vi "Clear Attachments2.vi"(0 "handles cluster in":T1 caption="ハンドルクラスター入力", 11 "error in (no error)":errorcluster caption="エラー入力（エラーなし）") -> (4 "handles cluster out":T1 caption="ハンドルクラスター出力", 15 "error out":errorcluster caption="エラー出力")   [LabVIEW 2015]
doc: "「Set Attachments2」VIを使用して設定したすべての添付を除去します。"
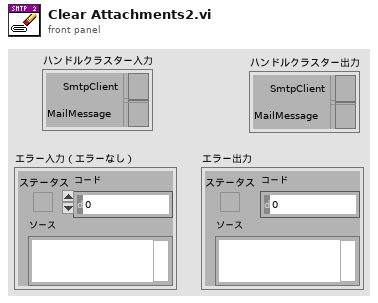
[diagram p1: front panel]
types:
  T1 = cluster{"SmtpClient":refnum<k24>, "MailMessage":refnum<k24>}
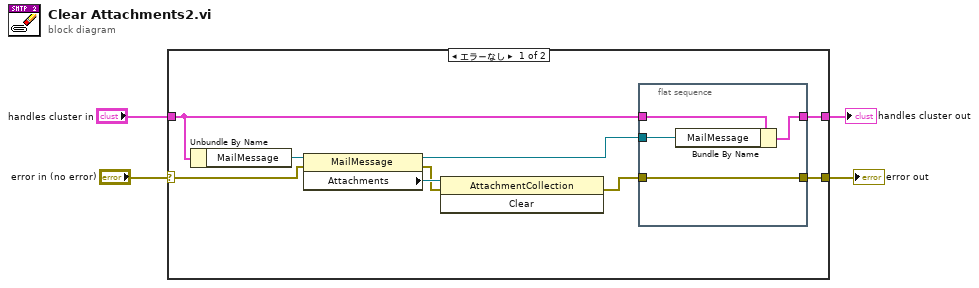
[diagram p0: block diagram]
diagram:
  n1 = case shown="エラーなし" "error in (no error)" {
    selector: "error in (no error)" -> [w10 w19]
    tunnel: [w6 w19] -> w3
    tunnel: "handles cluster in" -> [w13 w18]
    tunnel: [w12 w18] -> w1
    frame No Error {
      n2 = Unbundle By Name(w13) -> ("MailMessage"=w11:refnum<k24>)
      n3 = property class="MailMessage"(reference=w11, error in=w10) -> (reference out=w7:refnum<k24>, error out=w8:errorcluster, "Attachments"=w9:refnum<k24>)
      n4 = invoke class="AttachmentCollection" method="Clear"(reference=w9, error in=w8) -> (error out=w5:errorcluster)  [unwired: 1 in, 2 out]
      n5 = flat-sequence {
        tunnel: w13 -> [w17]
        tunnel: [w16] -> w12
        tunnel: w7 -> [w15]
        tunnel: w5 -> [w14]
        tunnel: [w14] -> w6
        frame #0 {
          n6 = Bundle By Name(cluster=w17, "MailMessage"=w15) -> (w16:T1)
        }
      }
    }
    frame Error {
    }
  }
  "handles cluster out" <- w1
  "error out" <- w3
